vi "Write Name.vi"(8 "error in (no error)":errorcluster, 10 "Name":string="csv", 11 "csv-formatter Config in":refnum<class "csv-formatter Config.lvclass">) -> (0 "error out":errorcluster, 3 "csv-formatter Config out":refnum<class "csv-formatter Config.lvclass">)   [LabVIEW 2015, in "csv-formatter Config.lvclass"]
uses:
  csv-formatter Config.lvclass
  csv-formatter Config.lvclass/csv-formatter Config.ctl
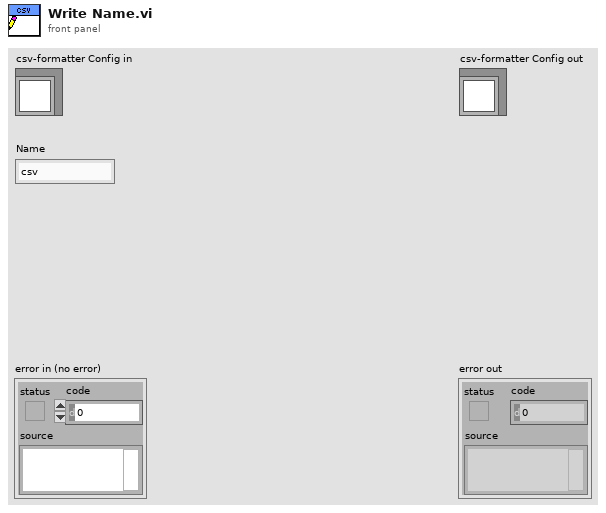
[diagram p1: front panel]
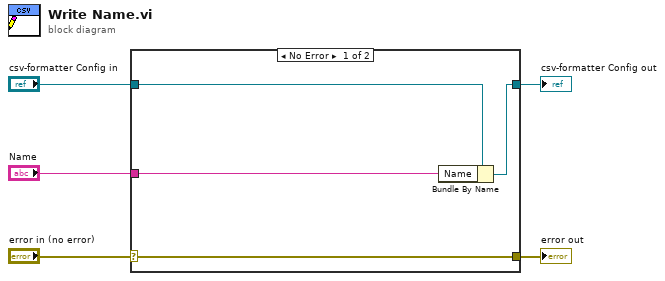
[diagram p0: block diagram]
diagram:
  n1 = case shown="No Error" "error in (no error)" {
    selector: "error in (no error)" -> [w9 w10]
    tunnel: [w9 w10] -> w4
    tunnel: [w7 w11] -> w2
    tunnel: "csv-formatter Config in" -> [w8 w11]
    tunnel: "Name" -> [w6 _]
    frame No Error {
      n2 = Bundle By Name(cluster=w8, "Name"=w6) -> (w7:refnum<class "csv-formatter Config.lvclass">)
    }
    frame Error {
    }
  }
  "error out" <- w4
  "csv-formatter Config out" <- w2
